vi "EXCEL 画曲线_210928.vi"(7 "自动化引用句柄":refnum<k7>, 8 "错误输入（无错误）":errorcluster, 11 "路径":path) -> (0 "error IO":errorcluster, 2 "XY图":cluster{"X":dbl, "Y":dbl}[](graph))   [LabVIEW 2018]
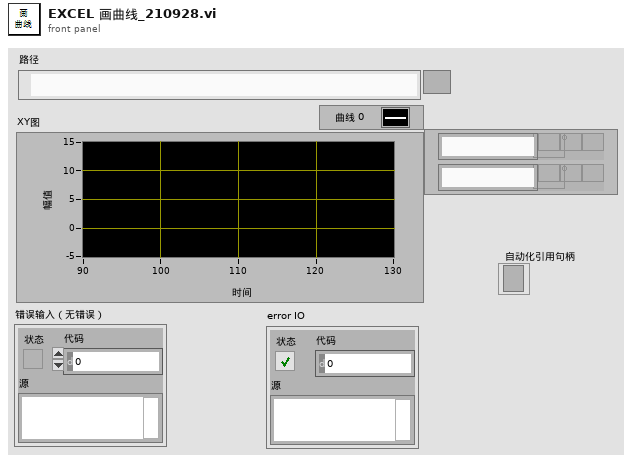
[diagram p1: front panel]
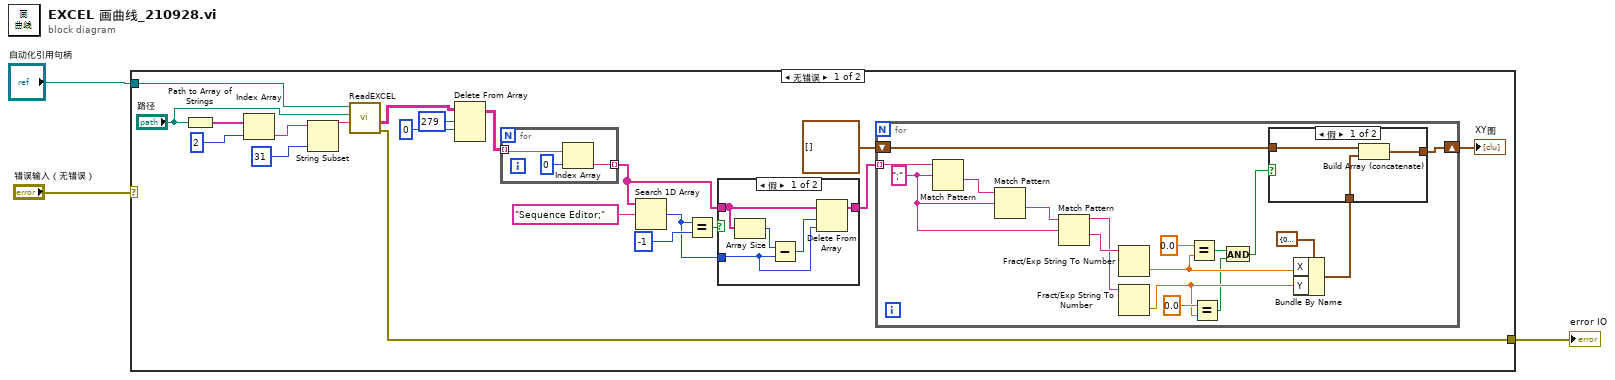
[diagram p0: block diagram]
diagram:
  n1 = case shown="无错误" "错误输入（无错误）" {
    selector: "错误输入（无错误）" -> [_ w54]
    tunnel: [w5 w54] -> w2
    tunnel: "自动化引用句柄" -> [w4 _]
    frame No Error {
      n2 = Path to Array of Strings(0:"路径") -> (2:w23:string[])  [unwired: 1 out]
      n3 = Index Array(array=w23, index=2 ("索引")) -> (element=w21:string)
      n4 = String Subset(string=w21, length (rest)=31 ("长度（剩余）")) -> (substring=w7:string)  [unwired: 1 in]
      n5 = call "ReadEXCEL.vi"("EXCEL 标签"=w7, "路径"="路径", "自动化引用句柄"=w4) -> ("错误输出"=w5:errorcluster, "数据"=w6:string[][])  [unwired: 7 in]
      n6 = Delete From Array(array=w6, length=279 ("长度"), index (row)=0 ("索引 (行)")) -> (array with subset deleted=w17:string[][])  [unwired: 1 in, 1 out]
      n7 = for {
        tunnel: w17 -> [w32] mode=indexing
        tunnel: [w30] -> w12 mode=indexing
        n8 = Index Array(array=w32, index=0 ("索引")) -> (element=w30:string)
      }
      n9 = Search 1D Array(1D array=w12, element="Sequence Editor;" ("元素")) -> (index of element=w9:i32)  [unwired: 1 in]
      n10 = Equal?(x=w9, y=-1) -> (x = y?=w10:bool)
      n11 = case shown="假" w10 {
        tunnel: w12 -> [w27 w29]
        tunnel: [w28 w29] -> w11
        tunnel: w9 -> [w24 _]
        frame False {
          n12 = Array Size(array=w27) -> (size(s)=w26:i32)
          n13 = Subtract(x=w26, y=w24) -> (x-y=w25:i32)
          n14 = Delete From Array(array=w27, length=w25, index=w24) -> (array with subset deleted=w28:string[])  [unwired: 1 out]
        }
        frame True {
        }
      }
      n15 = for {
        tunnel: w11 -> [w49] mode=indexing
        shift-right: [w33] -> w18
        shift-left: cluster{"X":dbl, "Y":dbl}[] [] ("XY图") -> [w45]
        w46 = ";" ("正则表达式")
        n16 = Match Pattern(string=w49, regular expression=w46) -> (after substring=w48:string)  [unwired: 1 in, 3 out]
        n17 = Match Pattern(string=w48, regular expression=w46) -> (after substring=w47:string)  [unwired: 1 in, 3 out]
        n18 = Match Pattern(string=w47, regular expression=w46) -> (before substring=w43:string, after substring=w44:string)  [unwired: 1 in, 2 out]
        n19 = Fract/Exp String To Number(string=w44) -> (number=w41:dbl)  [unwired: 3 in, 1 out]
        n20 = Fract/Exp String To Number(string=w43) -> (number=w38:dbl)  [unwired: 3 in, 1 out]
        n21 = Equal?(x=0.0, y=w41) -> (x = y?=w36:bool)
        n22 = Equal?(x=0.0, y=w38) -> (x = y?=w37:bool)
        n23 = And(x=w36, y=w37) -> (x .and. y?=w34:bool)
        n24 = Bundle By Name(cluster=cluster{"X":dbl, "Y":dbl} {"X"=0.0, "Y"=0.0}, "X"=w41, "Y"=w38) -> (w42:cluster{"X":dbl, "Y":dbl})
        n25 = case shown="假" w34 {
          tunnel: w45 -> [w52 w53]
          tunnel: [w51 w53] -> w33
          tunnel: w42 -> [w50 _]
          frame False {
            n26 = Build Array (concatenate)(w52, w50) -> (w51:cluster{"X":dbl, "Y":dbl}[])
          }
          frame True {
          }
        }
      }
      "XY图" <- w18
    }
    frame Error {
    }
  }
  "error IO" <- w2
